vi "Math-Subtract Mean.vi"(4 "Y":dbl[](array[numeric])) -> (1 "Y - mean(Y)":dbl[](array[numeric]))   [LabVIEW 2020]
uses:
  <vilib>/Analysis/baseanly.llb/Mean (DBL).vi
  <vilib>/Analysis/NI_AALBase.lvlib
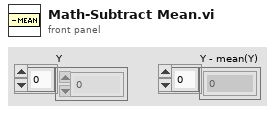
[diagram p1: front panel]
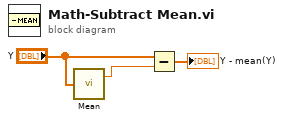
[diagram p0: block diagram]
diagram:
  n1 = call-poly <vilib>:"Mean.vi"("X"="Y") -> ("mean"=w2:dbl)  [unwired: 1 out]
  n2 = Subtract(x="Y", y=w2) -> (x-y=→"Y - mean(Y)":dbl[])
